vi "Barcode Print.vi"(6 "SN":string, 7 "Manual?":bool, 8 "error in":errorcluster, 9 "ECU Info":T1, 10 "Frame Barcode Formats":T2[](array[typedef]), 11 "part type":string) -> (0 "error out":errorcluster, 3 "SN out":string)   [LabVIEW 2018]
uses:
  typedefs/barcode format params.ctl
  typedefs/barcode printer types.ctl
  typedefs/open tcp connections.ctl
  <vilib>/Instr/_visa.llb/VISA Configure Serial Port (Instr).vi
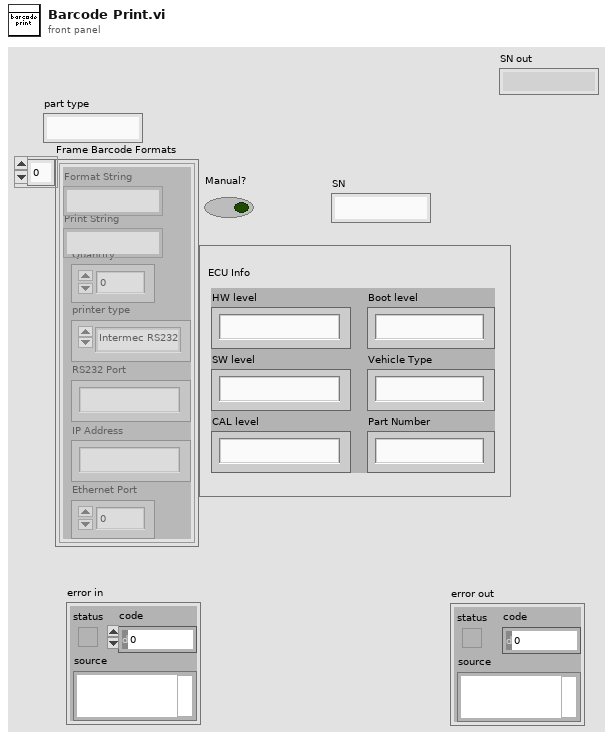
[diagram p1: front panel]
types:
  T1 = cluster{"HW level":string, "SW level":string, "CAL level":string, "Boot level":string, "Vehicle Type":string, "Part Number":string}
  T2 = typedef "barcode format params.ctl" = cluster{"Format String":string, "Print String":string, "Quantity":u8, "printer type":T3, "RS232 Port":string, "IP Address":string, "Ethernet Port":u32}
  T3 = typedef "barcode printer types.ctl" = enum16{"Intermec RS232", "Intermec Ethernet"}
  T4 = typedef "open tcp connections.ctl" = cluster{"ip address":string, "connection ID":refnum<k5>}
  T5 = cluster{"Frame Barcode Formats":T2[], "VISA resource name":refnum<visa-resource-name>, "Format String":string, "Print String":string, "Manual?":bool, "part type":string, "open rs232 ports":refnum<visa-resource-name>[], "open tcp ports":T4[], "to print":string[]}
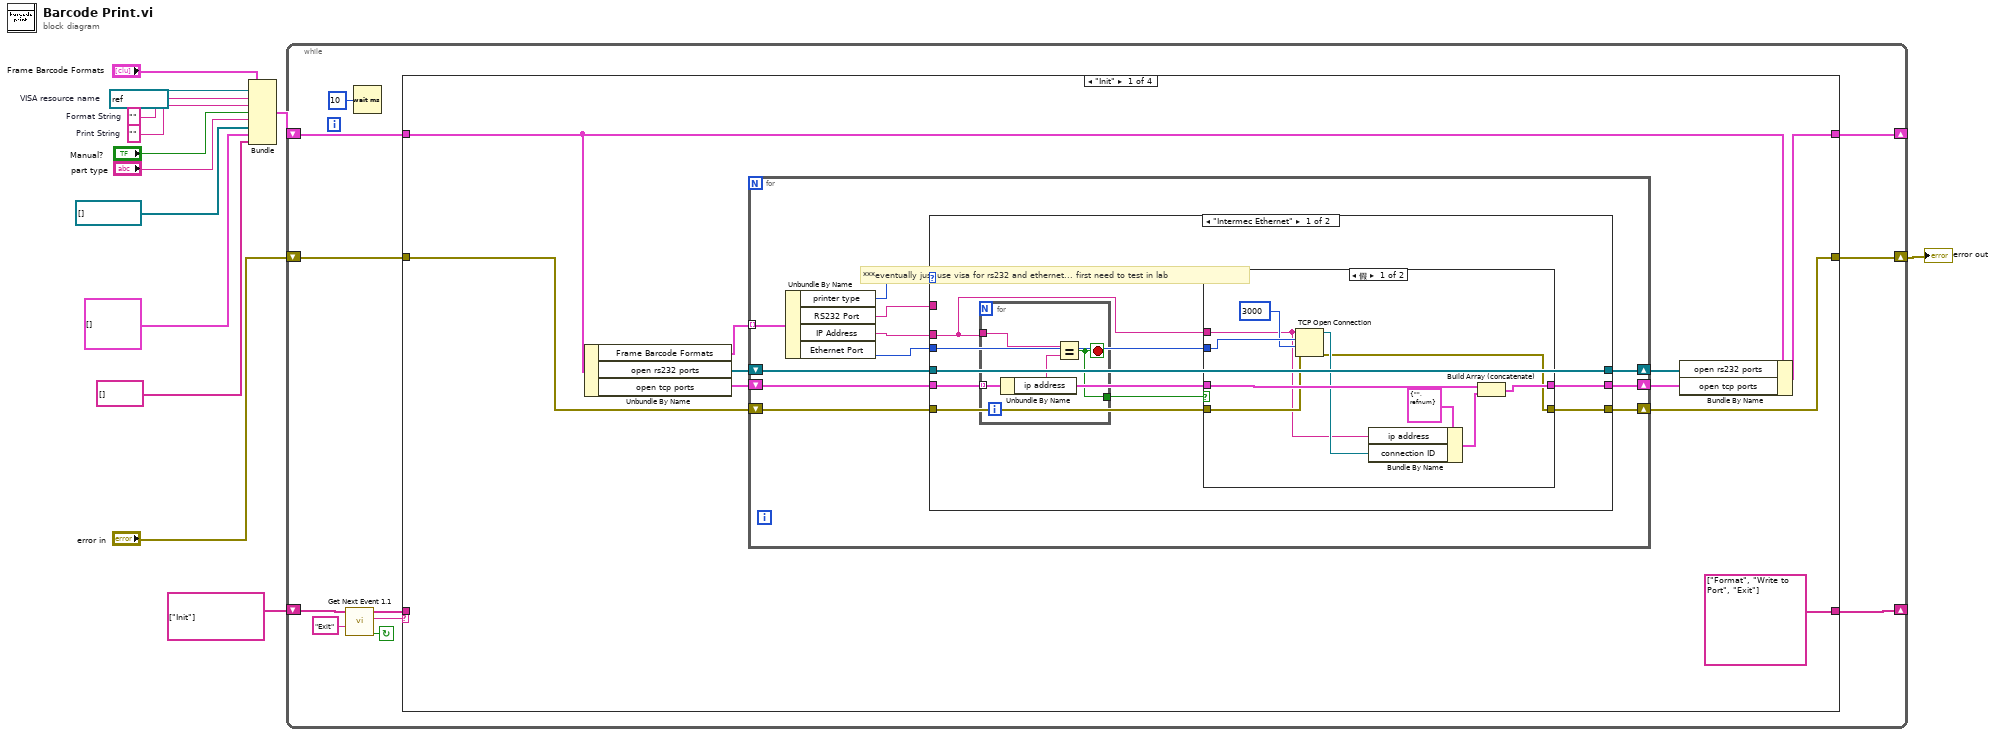
[diagram p0: block diagram]
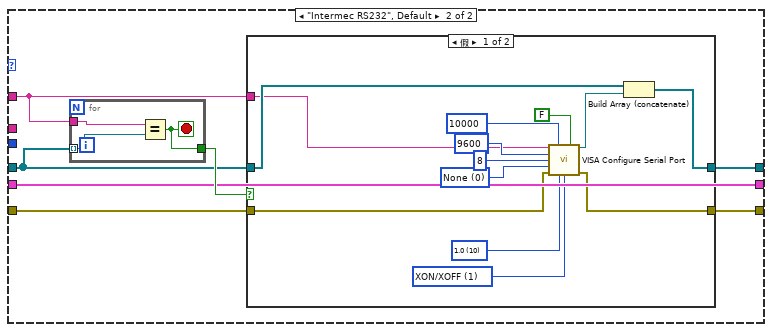
[diagram p3: hidden frame]
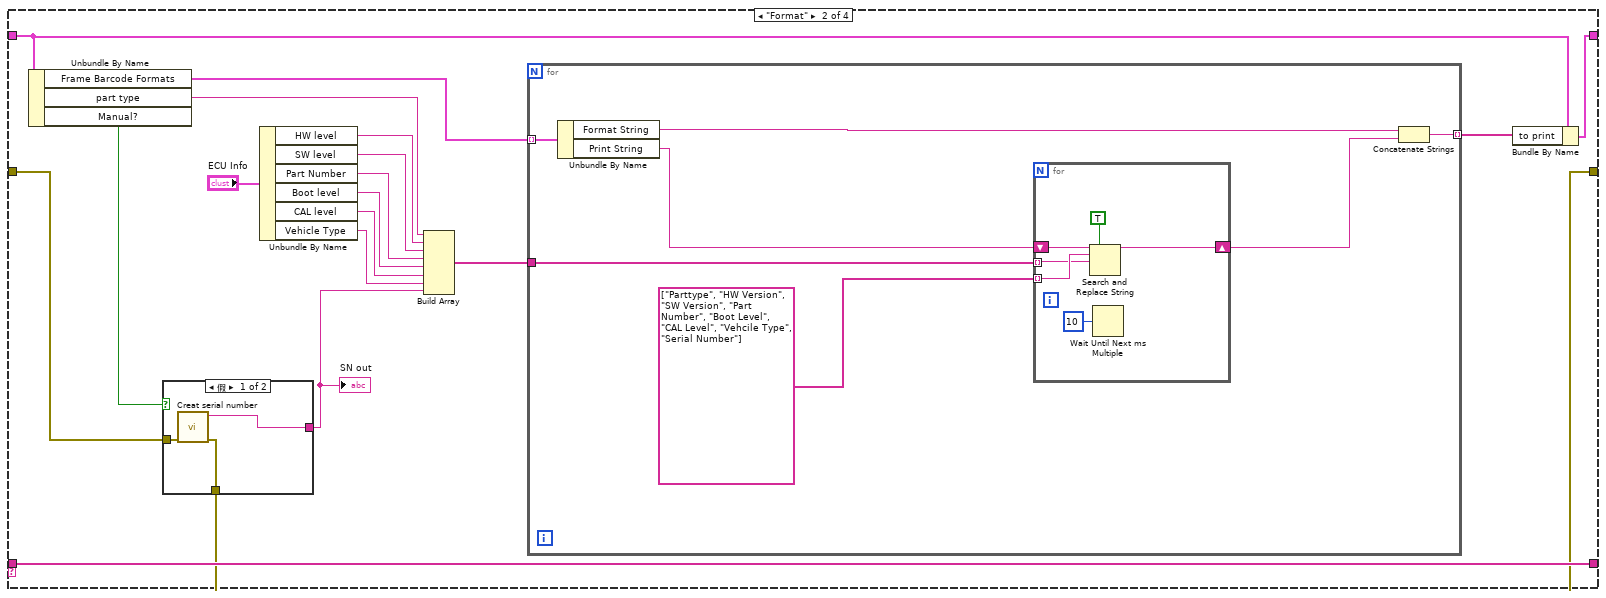
[diagram p5: hidden frame]
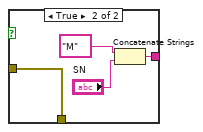
[diagram p6: hidden frame]
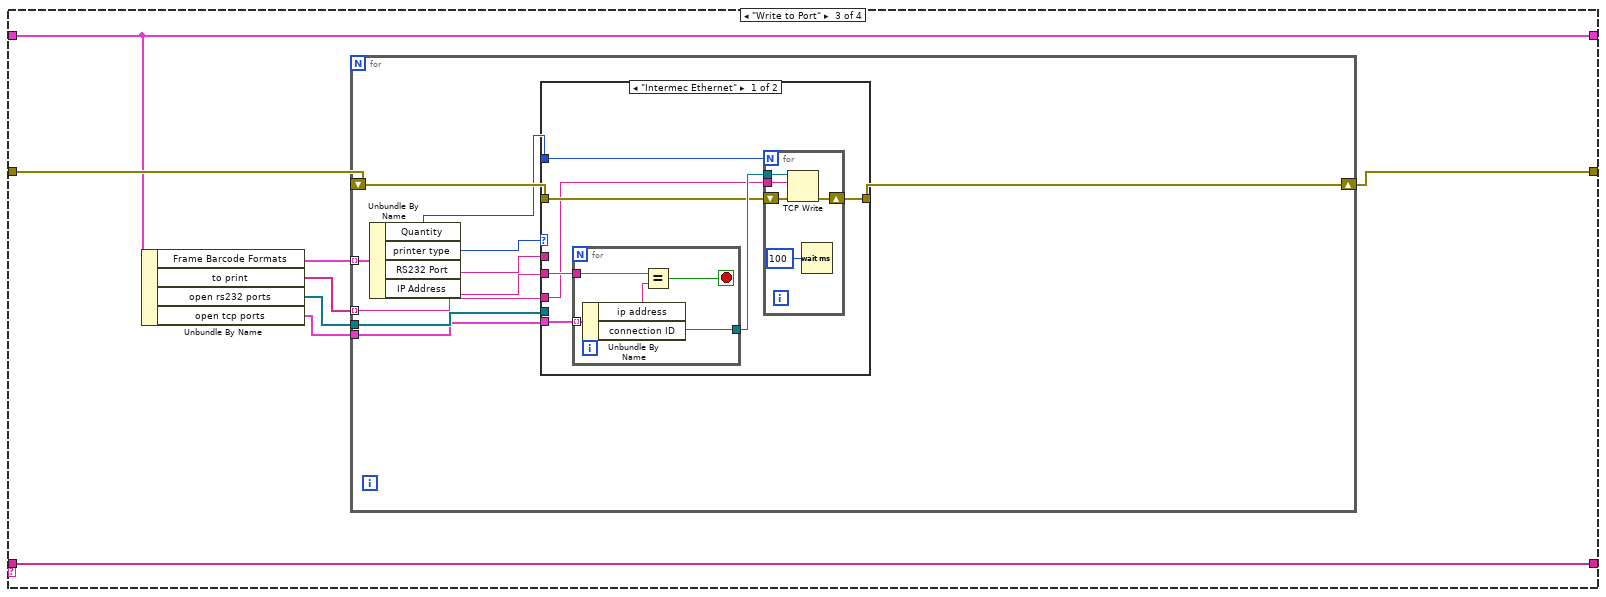
[diagram p7: hidden frame]
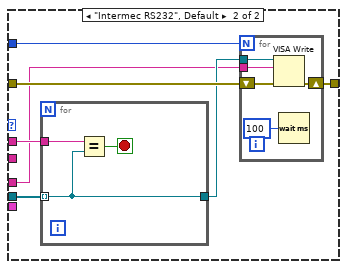
[diagram p8: hidden frame]
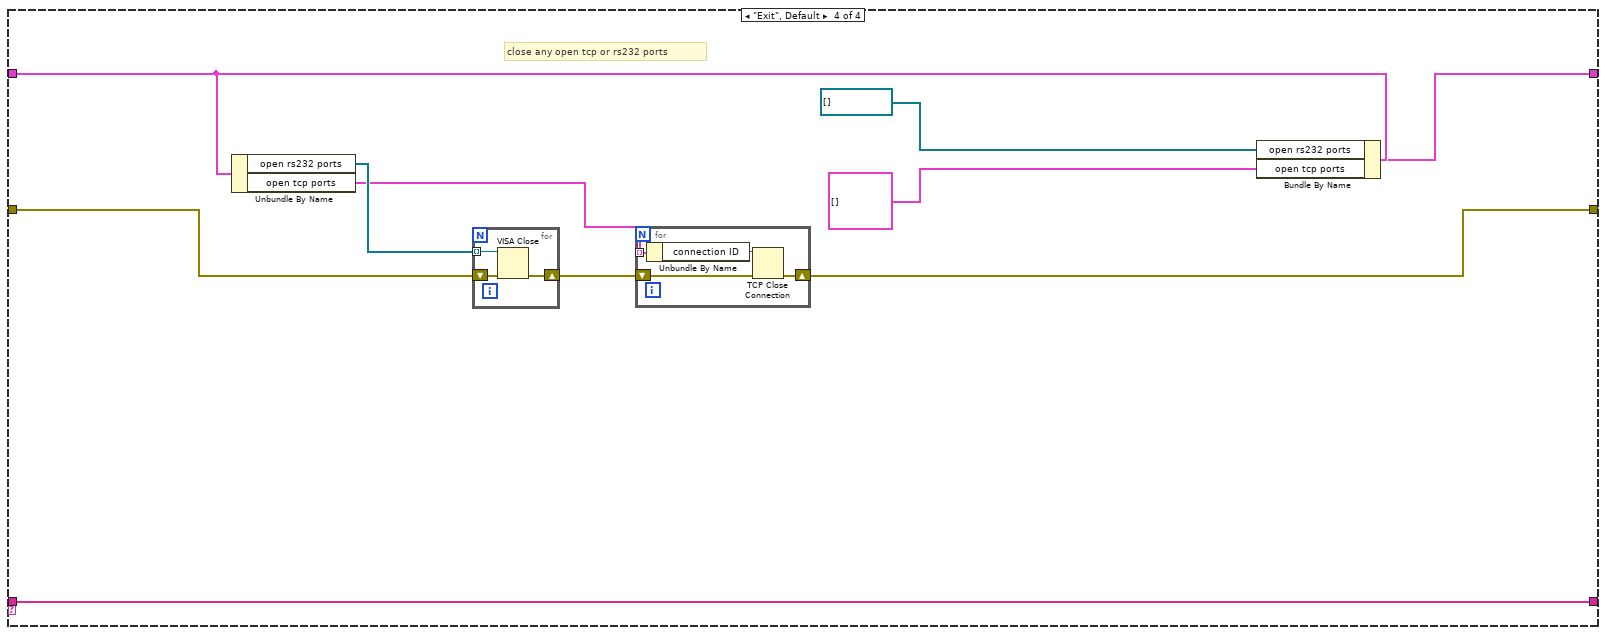
[diagram p9: hidden frame]
diagram:
  w10 = ""  # Print String
  w11 = refnum<visa-resource-name> "COM6"  # VISA resource name
  w12 = ""  # Format String
  n1 = Bundle("Frame Barcode Formats"="Frame Barcode Formats", "VISA resource name"=w11, "Format String"=w12, "Print String"=w10, "Manual?"="Manual?", "part type"="part type", "open rs232 ports"=refnum<visa-resource-name>[] [], "open tcp ports"=T4[] [], "to print"=string[] []) -> (w13:T5)  [unwired: 1 in]
  n2 = while {
    shift-right: [w22] -> _
    shift-left: string[] ["Init"] ("Event queue out") -> [w21]
    shift-right: [w18] -> _
    shift-left: w13 -> [w19]
    shift-right: [w14] -> w4
    shift-left: "error in" -> [w15]
    stop <- w20 continue-if-true
    n3 = call "Get Next Event 1.1.vi"("Exit Event"="Exit", "event queue in"=w21) -> ("Condition (Exit:F)"=w20:bool, "next event"=w24:string, "event queue out"=w23:string[])  [unwired: 6 in, 1 out]
    n4 = Wait (ms)(milliseconds to wait=u32 10) -> ()  [unwired: 1 out]
    n5 = case shown="\"Init\"" w24 {
      tunnel: w23 -> [_ w111 w139 w191]
      tunnel: [string[] ["Format", "Write to Port", "Exit"] ("event queue out") w111 w139 w191] -> w22
      tunnel: w19 -> [w32 w99 w136 w186]
      tunnel: [w34 w112 w136 w185] -> w18
      tunnel: w15 -> [w31 w102 w138 w190]
      tunnel: [w30 w101 w137 w188] -> w14
      frame "Init" {
        # "***eventually just use visa for rs232 and ethernet... first need to test in lab"
        n6 = Unbundle By Name(w32) -> ("Frame Barcode Formats"=w29:T2[], "open rs232 ports"=w28:refnum<visa-resource-name>[], "open tcp ports"=w27:T4[])
        n7 = for {
          tunnel: w29 -> [w45] mode=indexing
          shift-right: [w39] -> w26
          shift-left: w28 -> [w41]
          shift-right: [w40] -> w25
          shift-left: w27 -> [w42]
          shift-right: [w35] -> w30
          shift-left: w31 -> [w43]
          n8 = Unbundle By Name(w45) -> ("printer type"=w44:T3, "RS232 Port"=w38:string, "IP Address"=w37:string, "Ethernet Port"=w36:u32)
          n9 = case shown="\"Intermec Ethernet\"" w44 {
            tunnel: w43 -> [w47 w71]
            tunnel: w42 -> [w50 w75]
            tunnel: w41 -> [w53 w74]
            tunnel: [w51 w75] -> w40
            tunnel: [w53 w73] -> w39
            tunnel: w38 -> [_ w72]
            tunnel: w37 -> [w49 _]
            tunnel: w36 -> [w48 _]
            tunnel: [w46 w70] -> w35
            frame "Intermec Ethernet" {
              n10 = for {
                tunnel: w50 -> [w69] mode=indexing
                tunnel: w49 -> [w68]
                tunnel: [w66] -> w52
                stop <- w66 stop-if-true
                n11 = Unbundle By Name(w69) -> ("ip address"=w67:string)
                n12 = Equal?(x=w68, y=w67) -> (x = y?=w66:bool)
              }
              n13 = case shown="假" w52 {
                tunnel: [w60 w65] -> w51
                tunnel: w50 -> [w61 w65]
                tunnel: w49 -> [w54 _]
                tunnel: w48 -> [w63 _]
                tunnel: w47 -> [w56 w64]
                tunnel: [w55 w64] -> w46
                frame False {
                  n14 = TCP Open Connection(address=w54, remote port or service name=w63, timeout ms (60000)=3000, error in (no error)=w56) -> (connection ID=w57:refnum<k5>, error out=w55:errorcluster)  [unwired: 1 in]
                  n15 = Bundle By Name(cluster=T4 {"ip address"="", "connection ID"=refnum}, "ip address"=w54, "connection ID"=w57) -> (w58:T4)
                  n16 = Build Array (concatenate)(w61, w58) -> (w60:T4[])
                }
                frame True {
                }
              }
            }
            frame "Intermec RS232", Default {
              n17 = for {
                tunnel: w74 -> [w92] mode=indexing
                tunnel: w72 -> [w94]
                tunnel: [w93] -> w76
                stop <- w93 stop-if-true
                n18 = Equal?(x=w94, y=w92) -> (x = y?=w93:bool)
              }
              n19 = case shown="假" w76 {
                tunnel: w74 -> [w89 w91]
                tunnel: [w88 w91] -> w73
                tunnel: w72 -> [w80 _]
                tunnel: w71 -> [w78 w90]
                tunnel: [w77 w90] -> w70
                frame False {
                  w82 = u16 1 items=["None"=0, "XON/XOFF"=1, "RTS/CTS"=2, "DTR/DSR"=4] ("flow control")
                  w83 = u16 10 items=["1.0"=10, "1.5"=15, "2.0"=20] ("stop bits")
                  w86 = u16 0 items=["None", "Odd", "Even", "Mark", "Space"] ("parity")
                  n20 = call-poly "VISA Configure Serial Port"("VISA resource name"=w80, "timeout (10sec)"=u32 10000, "Enable Termination\nChar (T)"=FALSE ("Enable Termination Char (T)"), "baud rate (9600)"=u32 9600 ("baud rate"), "data bits (8)"=u16 8 ("data bits"), "parity (0:none)"=w86, "error in (no error)"=w78, "stop bits (10: 1 bit)"=w83, "flow control (0:none)"=w82) -> ("VISA resource name out"=w79:refnum<visa-resource-name>, "error out"=w77:errorcluster)  [unwired: 5 in]
                  n21 = Build Array (concatenate)(w89, w79) -> (w88:refnum<visa-resource-name>[])
                }
                frame True {
                }
              }
            }
          }
        }
        n22 = Bundle By Name(cluster=w32, "open rs232 ports"=w26, "open tcp ports"=w25) -> (w34:T5)
      }
      frame "Format" {
        n23 = Unbundle By Name(w99) -> ("Frame Barcode Formats"=w98:T2[], "part type"=w97:string, "Manual?"=w96:bool)
        n24 = case shown="假" w96 {
          tunnel: w102 -> [w115 w116]
          tunnel: [w114 w116] -> w101
          tunnel: [w113 w118] -> w95
          frame False {
            n25 = call "Creat serial number.vi"("error in (no error)"=w115) -> ("error out"=w114:errorcluster, "SN"=w113:string)  [unwired: 8 in, 1 out]
          }
          frame True {
            n26 = Concatenate Strings("M" ("string"), "SN") -> (w118:string)
          }
        }
        "SN out" <- w95
        n27 = Unbundle By Name("ECU Info") -> ("HW level"=w108:string, "SW level"=w107:string, "Part Number"=w106:string, "Boot level"=w105:string, "CAL level"=w104:string, "Vehicle Type"=w103:string)
        n28 = Build Array(w97, w108, w107, w106, w105, w104, w103, w95) -> (w100:string[])
        n29 = for {
          tunnel: [w126] -> w110 mode=indexing
          tunnel: w98 -> [w121] mode=indexing
          tunnel: w100 -> [w120]
          n30 = Unbundle By Name(w121) -> ("Format String"=w122:string, "Print String"=w125:string)
          n31 = for {
            shift-right: [w130] -> w123
            shift-left: w125 -> [w131]
            tunnel: string[] ["Parttype", "HW Version", "SW Version", "Part Number", "Boot Level", "CAL Level", "Vehcile Type", "Serial Number"] -> [w129] mode=indexing
            tunnel: w120 -> [w127] mode=indexing
            n32 = Search and Replace String(replace all?=TRUE ("replace all? (F)"), input string=w131, search string=w129, replace string=w127) -> (result string=w130:string)  [unwired: 4 in, 3 out]
            n33 = Wait Until Next ms Multiple(millisecond multiple=u32 10) -> ()  [unwired: 1 out]
          }
          n34 = Concatenate Strings(w122, w123) -> (w126:string)
        }
        n35 = Bundle By Name(cluster=w99, "to print"=w110) -> (w112:T5)
      }
      frame "Write to Port" {
        n36 = Unbundle By Name(w136) -> ("Frame Barcode Formats"=w140:T2[], "to print"=w135:string[], "open rs232 ports"=w134:refnum<visa-resource-name>[], "open tcp ports"=w133:T4[])
        n37 = for {
          shift-right: [w148] -> w137
          shift-left: w138 -> [w149]
          tunnel: w140 -> [w150] mode=indexing
          tunnel: w135 -> [w144] mode=indexing
          tunnel: w134 -> [w146]
          tunnel: w133 -> [w145]
          n38 = Unbundle By Name(w150) -> ("Quantity"=w141:u8, "printer type"=w143:T3, "RS232 Port"=w147:string, "IP Address"=w142:string)
          n39 = case shown="\"Intermec Ethernet\"" w143 {
            tunnel: w145 -> [w157 _]
            tunnel: w146 -> [_ w174]
            tunnel: w147 -> [_ w173]
            tunnel: w142 -> [w156 _]
            tunnel: w149 -> [w154 w172]
            tunnel: [w153 w171] -> w148
            tunnel: w144 -> [w152 w169]
            tunnel: w141 -> [w151 w168]
            frame "Intermec Ethernet" {
              n40 = for {
                tunnel: w157 -> [w167] mode=indexing
                tunnel: w156 -> [w166]
                tunnel: [w163] -> w155
                stop <- w164 stop-if-true
                n41 = Unbundle By Name(w167) -> ("ip address"=w165:string, "connection ID"=w163:refnum<k5>)
                n42 = Equal?(x=w166, y=w165) -> (x = y?=w164:bool)
              }
              n43 = for {
                N: w151 -> [_]
                tunnel: w155 -> [w162]
                tunnel: w152 -> [w159]
                shift-right: [w160] -> w153
                shift-left: w154 -> [w161]
                n44 = TCP Write(connection ID=w162, data in=w159, error in (no error)=w161) -> (error out=w160:errorcluster)  [unwired: 1 in, 2 out]
                n45 = Wait (ms)(milliseconds to wait=u32 100) -> ()  [unwired: 1 out]
              }
            }
            frame "Intermec RS232", Default {
              n46 = for {
                tunnel: w174 -> [w180] mode=indexing
                tunnel: w173 -> [w182]
                tunnel: [w180] -> w170
                stop <- w181 stop-if-true
                n47 = Equal?(x=w182, y=w180) -> (x = y?=w181:bool)
              }
              n48 = for {
                N: w168 -> [_]
                tunnel: w170 -> [w177]
                tunnel: w169 -> [w176]
                shift-right: [w178] -> w171
                shift-left: w172 -> [w179]
                n49 = VISA Write(VISA resource name=w177, write buffer=w176, error in (no error)=w179) -> (error out=w178:errorcluster)  [unwired: 2 out]
                n50 = Wait (ms)(milliseconds to wait=u32 100) -> ()  [unwired: 1 out]
              }
            }
          }
        }
      }
      frame "Exit", Default {
        # "close any open tcp or rs232 ports"
        n51 = Unbundle By Name(w186) -> ("open rs232 ports"=w192:refnum<visa-resource-name>[], "open tcp ports"=w187:T4[])
        n52 = for {
          tunnel: w192 -> [w199] mode=indexing
          shift-right: [w197] -> w189
          shift-left: w190 -> [w198]
          n53 = VISA Close(VISA resource name=w199, error in (no error)=w198) -> (error out=w197:errorcluster)
        }
        n54 = for {
          shift-right: [w195] -> w188
          shift-left: w189 -> [w196]
          tunnel: w187 -> [w194] mode=indexing
          n55 = Unbundle By Name(w194) -> ("connection ID"=w193:refnum<k5>)
          n56 = TCP Close Connection(connection ID=w193, error in (no error)=w196) -> (error out=w195:errorcluster)  [unwired: 1 in, 1 out]
        }
        n57 = Bundle By Name(cluster=w186, "open rs232 ports"=refnum<visa-resource-name>[] [], "open tcp ports"=T4[] []) -> (w185:T5)
      }
    }
  }
  "error out" <- w4
